vi "Register Enum Metadata.vi"(8 "error in":errorcluster, 10 "Enum Metadata":T2[](array[typedef]), 11 "gRPCid in":T1) -> (0 "error out":errorcluster, 3 "gRPCid out":T1)   [LabVIEW 2019, in "grpc-lvsupport.lvlib"]
uses:
  grpc-lvsupport.lvlib
  Enum Metadata.ctl
  grpcId.ctl
  <vilib>/Utility/file.llb/Application Directory.vi
  <vilib>/Utility/error.llb/Error Cluster From Error Code.vi
  <resource>/labview_grpc_server.dll
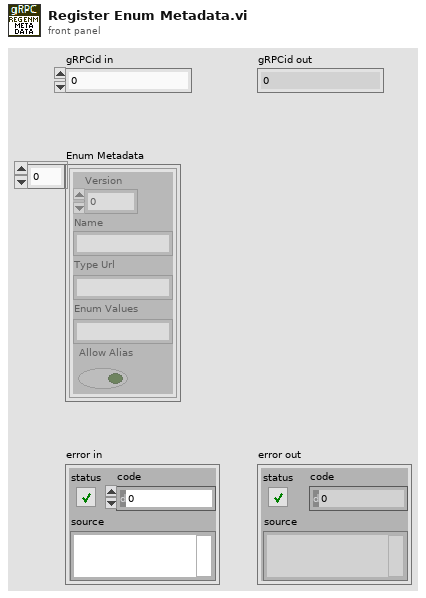
[diagram p1: front panel]
types:
  T1 = typedef "grpc-lvsupport.lvlib/grpcId.ctl" = u64
  T2 = typedef "grpc-lvsupport.lvlib/Enum Metadata.ctl" = cluster{"Version":i32, "Name":string, "Type Url":string, "Enum Values":string, "Allow Alias":bool}
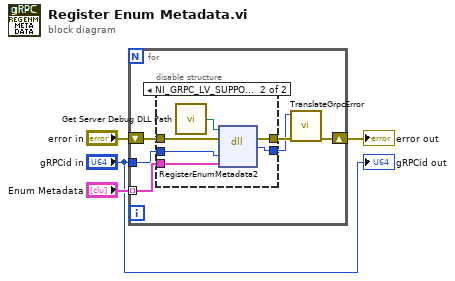
[diagram p0: block diagram]
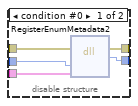
[diagram p2: hidden frame]
diagram:
  n1 = for {
    tunnel: "Enum Metadata" -> [w8] mode=indexing
    shift-right: [w6] -> w2
    shift-left: "error in" -> [w10]
    tunnel: "gRPCid in" -> [w7]
    n2 = disable-structure shown="NI_GRPC_LV_SUPPORT_DEBUG==True&&RUN_TIME_ENGINE==False" {
      disable-tunnel: w10 -> [w15 w21]
      disable-tunnel: [w14 w20] -> w9
      disable-tunnel: w8 -> [w13 w19]
      disable-tunnel: w7 -> [w12 w18]
      disable-tunnel: [w11 w17] -> w5
      frame condition #0 {
        n3 = dll-call lib="C:/Program Files (x86)/National Instruments/LabVIEW 2024/resource/labview_grpc_server.*" fn="RegisterEnumMetadata2"(error in=w15, "serverId"=w12, "metadata"=w13) -> (error out=w14:errorcluster, "return type"=w11:i32)  [unwired: 4 in, 1 out]
      }
      frame condition #1 (active) {
        n4 = call "Get Server Debug DLL Path.vi"() -> ("DLL Path"=w16:path)
        n5 = dll-call lib="?" fn="RegisterEnumMetadata2"(path in=w16, error in=w21, "serverId"=w18, "metadata"=w19) -> (error out=w20:errorcluster, "return type"=w17:i32)  [unwired: 3 in, 1 out]
      }
    }
    n6 = call "TranslateGrpcError.vi"("error in"=w9, "Error Code"=w5) -> ("error out"=w6:errorcluster)  [unwired: 9 in]
  }
  "error out" <- w2
  "gRPCid out" <- "gRPCid in"
